vi "Mercury_GoToField_SubVI.vi"(8 "error in (no error)":errorcluster, 11 "Mercury Targets":T1) -> (0 "error out":errorcluster)   [LabVIEW 2016]
doc: "USE AT YOUR OWN RISK!\nThis subVI is meant to be called as a subVI of \"Mercury_GoToField.vi\", which will take care of the persistent switch for you"
panel:
  # "USE AT YOUR OWN RISK!\nThis subVI is meant to be called as a subVI of \"Mercury_GoToField.vi\", which will take care of the persistent switch for you"
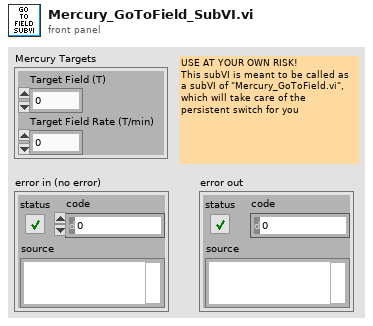
[diagram p1: front panel]
types:
  T1 = cluster{"Target Field (T)":dbl, "Target Field Rate (T/min)":dbl}
  T2 = cluster{"Hold":bool, "Clamp":bool, "To Set":bool, "To Zero":bool, "Send to IPS":bool, "PS Heat":bool, "Lambda":bool}
  T3 = cluster{"Magnet Field":dbl, "PS Field":dbl, "Target Field":dbl, "Target Field Rate":dbl, "Voltage":dbl, "Current":dbl, "Switch":bool}
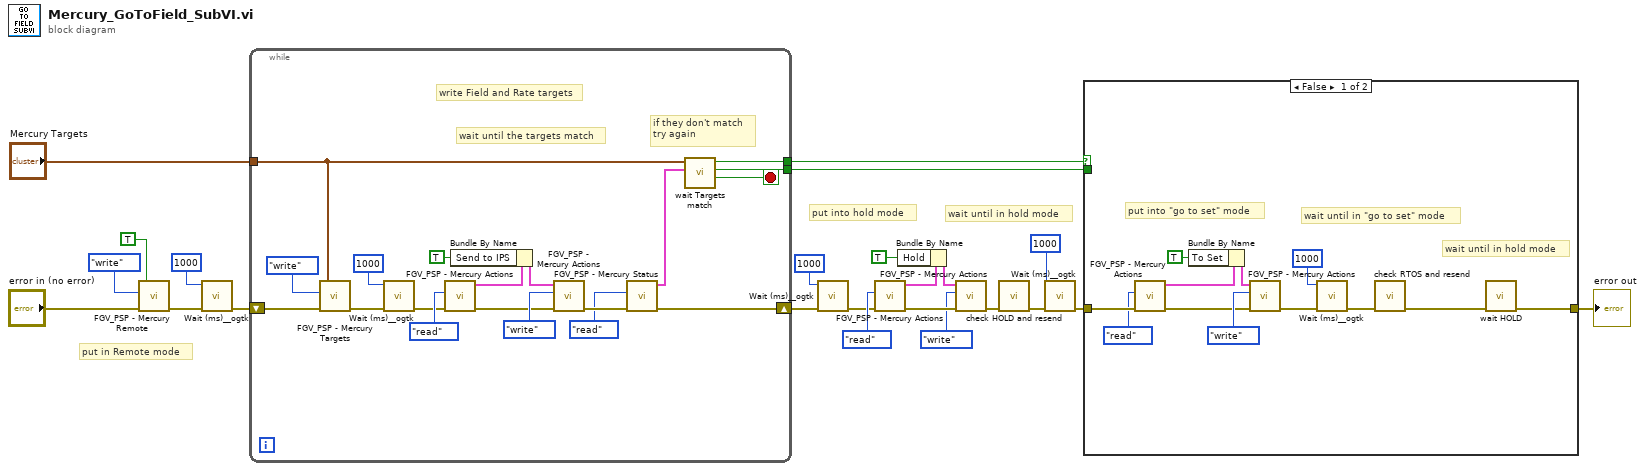
[diagram p0: block diagram]
diagram:
  # "put in Remote mode"
  # "wait until in hold mode"
  # "put into hold mode"
  n1 = call "FGV_PSP - Mercury Remote.vi"("error in"="error in (no error)", "Function"=enum16{"write", "read"}."write", "Mercury Remote"=TRUE) -> ("error out"=w9:errorcluster)  [unwired: 3 in, 1 out]
  n2 = call <userlib>:"Wait (ms)__ogtk.vi"("error in (no error)"=w9, "milliseconds to wait"=u32 1000) -> ("error out"=w8:errorcluster)  [unwired: 8 in, 1 out]
  n3 = while {
    tunnel: "Mercury Targets" -> [w42]
    tunnel: [w25] -> w18
    tunnel: [w38] -> w17
    shift-right: [w37] -> w16
    shift-left: w8 -> [w39]
    stop <- w35 stop-if-true
    # "if they don't match\ntry again"
    # "wait until the targets match"
    # "write Field and Rate targets"
    n4 = call "FGV_PSP - Mercury Targets.vi"("error in"=w39, "Function"=enum16{"write", "read"}."write", "Mercury Targets"=w42) -> ("error out"=w33:errorcluster)  [unwired: 3 in, 1 out]
    n5 = call <userlib>:"Wait (ms)__ogtk.vi"("error in (no error)"=w33, "milliseconds to wait"=u32 1000) -> ("error out"=w29:errorcluster)  [unwired: 8 in, 1 out]
    n6 = call "FGV_PSP - Mercury Actions.vi"("error in"=w29, "Function"=enum16{"write", "read"}."read") -> ("error out"=w28:errorcluster, "mercury actions 2"=w27:T2)  [unwired: 4 in]
    n7 = Bundle By Name(cluster=w27, "Send to IPS"=TRUE) -> (w26:T2)
    n8 = call "FGV_PSP - Mercury Actions.vi"("error in"=w28, "Function"=enum16{"write", "read"}."write", "mercury actions"=w26) -> ("error out"=w41:errorcluster)  [unwired: 3 in, 1 out]
    n9 = call "FGV_PSP - Mercury Status.vi"("error in"=w41, "Function"=enum16{"write", "read"}."read") -> ("error out"=w37:errorcluster, "status"=w24:T3)  [unwired: 4 in]
    n10 = call "wait Targets match.vi"("status"=w24, "Mercury Targets"=w42) -> ("Target AND Rate Match"=w35:bool, "Target ~ Magnet"=w38:bool, "Target ~ PS"=w25:bool)  [unwired: 7 in]
  }
  n11 = call <userlib>:"Wait (ms)__ogtk.vi"("error in (no error)"=w16, "milliseconds to wait"=u32 1000) -> ("error out"=w5:errorcluster)  [unwired: 8 in, 1 out]
  n12 = call "FGV_PSP - Mercury Actions.vi"("error in"=w5, "Function"=enum16{"write", "read"}."read") -> ("error out"=w4:errorcluster, "mercury actions 2"=w3:T2)  [unwired: 4 in]
  n13 = Bundle By Name(cluster=w3, "Hold"=TRUE ("Send to IPS")) -> (w2:T2)
  n14 = call "FGV_PSP - Mercury Actions.vi"("error in"=w4, "Function"=enum16{"write", "read"}."write", "mercury actions"=w2) -> ("error out"=w12:errorcluster)  [unwired: 3 in, 1 out]
  n15 = call "check HOLD and resend.vi"("error in"=w12) -> ("error out 2"=w11:errorcluster)  [unwired: 10 in]
  n16 = call <userlib>:"Wait (ms)__ogtk.vi"("error in (no error)"=w11, "milliseconds to wait"=u32 1000) -> ("error out"=w14:errorcluster)  [unwired: 8 in, 1 out]
  n17 = case shown="False" w18 {
    tunnel: [w54 w55] -> w23
    tunnel: w14 -> [w46 w55]
    tunnel: w17 -> [_ _]
    frame False {
      # "put into \"go to set\" mode"
      # "wait until in hold mode"
      # "wait until in \"go to set\" mode"
      n18 = call "FGV_PSP - Mercury Actions.vi"("error in"=w46, "Function"=enum16{"write", "read"}."read") -> ("error out"=w44:errorcluster, "mercury actions 2"=w45:T2)  [unwired: 4 in]
      n19 = Bundle By Name(cluster=w45, "To Set"=TRUE ("Send to IPS")) -> (w47:T2)
      n20 = call "FGV_PSP - Mercury Actions.vi"("error in"=w44, "Function"=enum16{"write", "read"}."write", "mercury actions"=w47) -> ("error out"=w50:errorcluster)  [unwired: 3 in, 1 out]
      n21 = call <userlib>:"Wait (ms)__ogtk.vi"("error in (no error)"=w50, "milliseconds to wait"=u32 1000) -> ("error out"=w49:errorcluster)  [unwired: 8 in, 1 out]
      n22 = call "check RTOS and resend.vi"("error in"=w49) -> ("error out 2"=w48:errorcluster)  [unwired: 10 in]
      n23 = call "wait HOLD.vi"("error in (no error)"=w48) -> ("error out"=w54:errorcluster)  [unwired: 10 in]
    }
    frame True {
      # "if Target Field = Power Supply Field do not\nput into \"Go To Set\" mode"
    }
  }
  "error out" <- w23
